vi "CHR12061 DMM Main.vi"   [LabVIEW 2018]
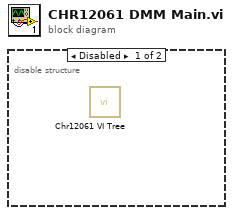
[diagram p0: block diagram]
diagram:
  n1 = disable-structure shown="Disabled" {
    frame Disabled {
      n2 = call <instrlib>:"Chr12061 VI Tree.vi"() -> ()  [unwired: 12 in]
    }
    frame Enabled {
    }
  }
